vi "CIMAQ_GetPalette.vi"(8 "error in":errorcluster, 11 "Palette Number (gray)":T1(ring)=enum."Full Rainbow") -> (0 "error out":errorcluster, 3 "User Palette":cluster{"Red":u8, "Green":u8, "Blue":u8}[](array[cluster]))   [LabVIEW 2017]
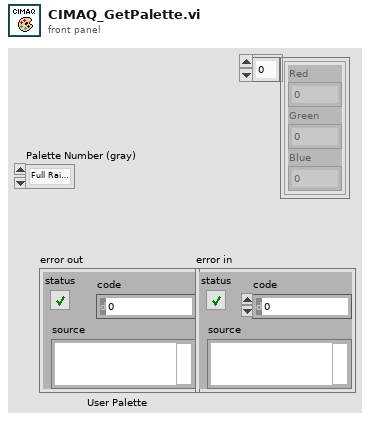
[diagram p1: front panel]
types:
  T1 = enum32{"Gray", "Binary", "Gradient", "Rainbow", "Temperature", "Full Rainbow", "Iron", "Hot Iron", "Hot Metal Blue", "PET"}
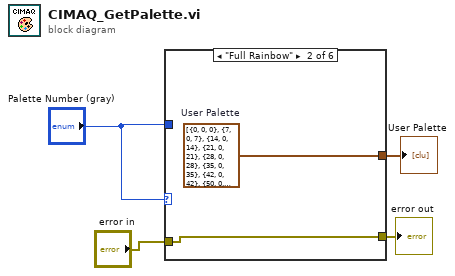
[diagram p0: block diagram]
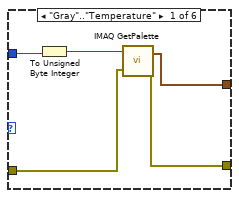
[diagram p2: hidden frame]
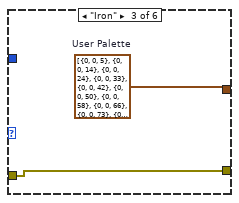
[diagram p3: hidden frame]
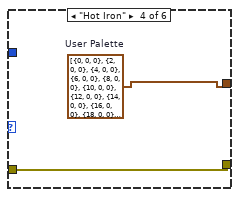
[diagram p4: hidden frame]
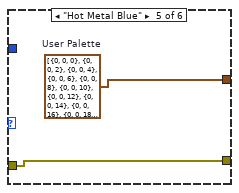
[diagram p5: hidden frame]
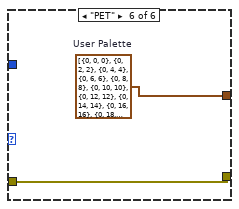
[diagram p6: hidden frame]
diagram:
  n1 = case shown="\"Full Rainbow\"" "Palette Number (gray)" {
    tunnel: "Palette Number (gray)" -> [w9 _ _ _ _ _]
    tunnel: [w7 w11 w13 w14 w17 w18] -> w1
    tunnel: [w6 w10 w12 w15 w16 w19] -> w3
    tunnel: "error in" -> [w5 w10 w12 w15 w16 w19]
    frame "Gray".."Temperature" {
      n2 = To Unsigned Byte Integer(number=w9) -> (unsigned 8bit integer=w8:u8)
      n3 = call "IMAQ GetPalette"("Palette Number (gray)"=w8, "error in (no error)"=w5) -> ("Color Palette"=w7:cluster{"Red":u8, "Green":u8, "Blue":u8}[], "error out"=w6:errorcluster)  [unwired: 3 in]
    }
    frame "Full Rainbow" {
      w11 = cluster{"Red":u8, "Green":u8, "Blue":u8}[] [{"Red"=0, "Green"=0, "Blue"=0}, {"Red"=7, "Green"=0, "Blue"=7}, {"Red"=14, "Green"=0, "Blue"=14}, {"Red"=21, "Green"=0, "Blue"=21}, {"Red"=28, "Green"=0, "Blue"=28}, {"Red"=35, "Green"=0, "Blue"=35}, {"Red"=42, "Green"=0, "Blue"=42}, {"Red"=50, "Green"=0, "Blue"=50}, {"Red"=57, "Green"=0, "Blue"=57}, {"Red"=64, "Green"=0, "Blue"=64}, {"Red"=71, "Green"=0, "Blue"=71}, {"Red"=78, "Green"=0, "Blue"=78}, {"Red"=85, "Green"=0, "Blue"=85}, {"Red"=92, "Green"=0, "Blue"=92}, {"Red"=99, "Green"=0, "Blue"=99}, {"Red"=106, "Green"=0, "Blue"=106}, {"Red"=113, "Green"=0, "Blue"=113}, {"Red"=120, "Green"=0, "Blue"=120}, {"Red"=128, "Green"=0, "Blue"=128}, {"Red"=135, "Green"=0, "Blue"=135}, {"Red"=142, "Green"=0, "Blue"=142}, {"Red"=149, "Green"=0, "Blue"=149}, {"Red"=156, "Green"=0, "Blue"=156}, {"Red"=163, "Green"=0, "Blue"=163}, {"Red"=170, "Green"=0, "Blue"=170}, {"Red"=177, "Green"=0, "Blue"=177}, {"Red"=184, "Green"=0, "Blue"=184}, {"Red"=191, "Green"=0, "Blue"=191}, {"Red"=198, "Green"=0, "Blue"=198}, {"Red"=205, "Green"=0, "Blue"=205}, {"Red"=212, "Green"=0, "Blue"=212}, {"Red"=220, "Green"=0, "Blue"=220}, {"Red"=227, "Green"=0, "Blue"=227}, {"Red"=234, "Green"=0, "Blue"=234}, {"Red"=241, "Green"=0, "Blue"=241}, {"Red"=248, "Green"=0, "Blue"=248}, {"Red"=255, "Green"=0, "Blue"=255}, {"Red"=248, "Green"=0, "Blue"=253}, {"Red"=241, "Green"=0, "Blue"=251}, {"Red"=234, "Green"=0, "Blue"=249}, {"Red"=227, "Green"=0, "Blue"=247}, {"Red"=220, "Green"=0, "Blue"=245}, {"Red"=212, "Green"=0, "Blue"=242}, {"Red"=205, "Green"=0, "Blue"=240}, {"Red"=198, "Green"=0, "Blue"=238}, {"Red"=191, "Green"=0, "Blue"=236}, {"Red"=184, "Green"=0, "Blue"=234}, {"Red"=177, "Green"=0, "Blue"=232}, {"Red"=170, "Green"=0, "Blue"=230}, {"Red"=163, "Green"=0, "Blue"=228}, {"Red"=156, "Green"=0, "Blue"=226}, {"Red"=149, "Green"=0, "Blue"=224}, {"Red"=142, "Green"=0, "Blue"=222}, {"Red"=135, "Green"=0, "Blue"=220}, {"Red"=128, "Green"=0, "Blue"=218}, {"Red"=120, "Green"=0, "Blue"=215}, {"Red"=113, "Green"=0, "Blue"=213}, {"Red"=106, "Green"=0, "Blue"=211}, {"Red"=99, "Green"=0, "Blue"=209}, {"Red"=92, "Green"=0, "Blue"=207}, {"Red"=85, "Green"=0, "Blue"=205}, {"Red"=78, "Green"=0, "Blue"=203}, {"Red"=71, "Green"=0, "Blue"=201}, {"Red"=64, "Green"=0, "Blue"=199}, {"Red"=57, "Green"=0, "Blue"=197}, {"Red"=50, "Green"=0, "Blue"=195}, {"Red"=42, "Green"=0, "Blue"=192}, {"Red"=35, "Green"=0, "Blue"=190}, {"Red"=28, "Green"=0, "Blue"=188}, {"Red"=21, "Green"=0, "Blue"=186}, {"Red"=14, "Green"=0, "Blue"=184}, {"Red"=7, "Green"=0, "Blue"=182}, {"Red"=0, "Green"=0, "Blue"=180}, {"Red"=0, "Green"=7, "Blue"=182}, {"Red"=0, "Green"=14, "Blue"=184}, {"Red"=0, "Green"=21, "Blue"=186}, {"Red"=0, "Green"=28, "Blue"=188}, {"Red"=0, "Green"=35, "Blue"=190}, {"Red"=0, "Green"=42, "Blue"=192}, {"Red"=0, "Green"=50, "Blue"=194}, {"Red"=0, "Green"=57, "Blue"=196}, {"Red"=0, "Green"=64, "Blue"=198}, {"Red"=0, "Green"=71, "Blue"=201}, {"Red"=0, "Green"=78, "Blue"=203}, {"Red"=0, "Green"=85, "Blue"=205}, {"Red"=0, "Green"=92, "Blue"=207}, {"Red"=0, "Green"=99, "Blue"=209}, {"Red"=0, "Green"=106, "Blue"=211}, {"Red"=0, "Green"=113, "Blue"=213}, {"Red"=0, "Green"=120, "Blue"=215}, {"Red"=0, "Green"=128, "Blue"=217}, {"Red"=0, "Green"=135, "Blue"=219}, {"Red"=0, "Green"=142, "Blue"=221}, {"Red"=0, "Green"=149, "Blue"=223}, {"Red"=0, "Green"=156, "Blue"=225}, {"Red"=0, "Green"=163, "Blue"=227}, {"Red"=0, "Green"=170, "Blue"=229}, {"Red"=0, "Green"=177, "Blue"=231}, {"Red"=0, "Green"=184, "Blue"=233}, {"Red"=0, "Green"=191, "Blue"=236}, {"Red"=0, "Green"=198, "Blue"=238}, {"Red"=0, "Green"=205, "Blue"=240}, {"Red"=0, "Green"=213, "Blue"=242}, {"Red"=0, "Green"=220, "Blue"=244}, {"Red"=0, "Green"=227, "Blue"=246}, {"Red"=0, "Green"=234, "Blue"=248}, {"Red"=0, "Green"=241, "Blue"=250}, {"Red"=0, "Green"=248, "Blue"=252}, {"Red"=0, "Green"=255, "Blue"=254}, {"Red"=0, "Green"=253, "Blue"=247}, {"Red"=0, "Green"=251, "Blue"=240}, {"Red"=0, "Green"=250, "Blue"=233}, {"Red"=0, "Green"=248, "Blue"=226}, {"Red"=0, "Green"=246, "Blue"=219}, {"Red"=0, "Green"=244, "Blue"=212}, {"Red"=0, "Green"=242, "Blue"=205}, {"Red"=0, "Green"=241, "Blue"=198}, {"Red"=0, "Green"=239, "Blue"=190}, {"Red"=0, "Green"=237, "Blue"=183}, {"Red"=0, "Green"=235, "Blue"=176}, {"Red"=0, "Green"=233, "Blue"=169}, {"Red"=0, "Green"=232, "Blue"=162}, {"Red"=0, "Green"=230, "Blue"=155}, {"Red"=0, "Green"=228, "Blue"=148}, {"Red"=0, "Green"=226, "Blue"=141}, {"Red"=0, "Green"=224, "Blue"=134}, {"Red"=0, "Green"=222, "Blue"=127}, {"Red"=0, "Green"=221, "Blue"=120}, {"Red"=0, "Green"=219, "Blue"=113}, {"Red"=0, "Green"=217, "Blue"=106}, {"Red"=0, "Green"=215, "Blue"=99}, {"Red"=0, "Green"=213, "Blue"=92}, {"Red"=0, "Green"=212, "Blue"=85}, {"Red"=0, "Green"=210, "Blue"=78}, {"Red"=0, "Green"=208, "Blue"=71}, {"Red"=0, "Green"=206, "Blue"=64}, {"Red"=0, "Green"=204, "Blue"=56}, {"Red"=0, "Green"=203, "Blue"=49}, {"Red"=0, "Green"=201, "Blue"=42}, {"Red"=0, "Green"=199, "Blue"=35}, {"Red"=0, "Green"=197, "Blue"=28}, {"Red"=0, "Green"=195, "Blue"=21}, {"Red"=0, "Green"=194, "Blue"=14}, {"Red"=0, "Green"=192, "Blue"=7}, {"Red"=0, "Green"=190, "Blue"=0}, {"Red"=7, "Green"=192, "Blue"=0}, {"Red"=14, "Green"=194, "Blue"=0}, {"Red"=21, "Green"=195, "Blue"=0}, {"Red"=28, "Green"=197, "Blue"=0}, {"Red"=35, "Green"=199, "Blue"=0}, {"Red"=43, "Green"=201, "Blue"=0}, {"Red"=50, "Green"=202, "Blue"=0}, {"Red"=57, "Green"=204, "Blue"=0}, {"Red"=64, "Green"=206, "Blue"=0}, {"Red"=71, "Green"=208, "Blue"=0}, {"Red"=78, "Green"=210, "Blue"=0}, {"Red"=85, "Green"=211, "Blue"=0}, {"Red"=92, "Green"=213, "Blue"=0}, {"Red"=99, "Green"=215, "Blue"=0}, {"Red"=106, "Green"=217, "Blue"=0}, {"Red"=113, "Green"=218, "Blue"=0}, {"Red"=120, "Green"=220, "Blue"=0}, {"Red"=128, "Green"=222, "Blue"=0}, {"Red"=135, "Green"=224, "Blue"=0}, {"Red"=142, "Green"=226, "Blue"=0}, {"Red"=149, "Green"=227, "Blue"=0}, {"Red"=156, "Green"=229, "Blue"=0}, {"Red"=163, "Green"=231, "Blue"=0}, {"Red"=170, "Green"=233, "Blue"=0}, {"Red"=177, "Green"=234, "Blue"=0}, {"Red"=184, "Green"=236, "Blue"=0}, {"Red"=191, "Green"=238, "Blue"=0}, {"Red"=198, "Green"=240, "Blue"=0}, {"Red"=205, "Green"=242, "Blue"=0}, {"Red"=212, "Green"=243, "Blue"=0}, {"Red"=220, "Green"=245, "Blue"=0}, {"Red"=227, "Green"=247, "Blue"=0}, {"Red"=234, "Green"=249, "Blue"=0}, {"Red"=241, "Green"=250, "Blue"=0}, {"Red"=248, "Green"=252, "Blue"=0}, {"Red"=255, "Green"=254, "Blue"=0}, {"Red"=253, "Green"=247, "Blue"=0}, {"Red"=252, "Green"=240, "Blue"=0}, {"Red"=250, "Green"=233, "Blue"=0}, {"Red"=249, "Green"=226, "Blue"=0}, {"Red"=247, "Green"=219, "Blue"=0}, {"Red"=246, "Green"=212, "Blue"=0}, {"Red"=244, "Green"=205, "Blue"=0}, {"Red"=243, "Green"=198, "Blue"=0}, {"Red"=241, "Green"=190, "Blue"=0}, {"Red"=239, "Green"=183, "Blue"=0}, {"Red"=238, "Green"=176, "Blue"=0}, {"Red"=236, "Green"=169, "Blue"=0}, {"Red"=235, "Green"=162, "Blue"=0}, {"Red"=233, "Green"=155, "Blue"=0}, {"Red"=232, "Green"=148, "Blue"=0}, {"Red"=230, "Green"=141, "Blue"=0}, {"Red"=229, "Green"=134, "Blue"=0}, {"Red"=227, "Green"=127, "Blue"=0}, {"Red"=225, "Green"=120, "Blue"=0}, {"Red"=224, "Green"=113, "Blue"=0}, {"Red"=222, "Green"=106, "Blue"=0}, {"Red"=221, "Green"=99, "Blue"=0}, {"Red"=219, "Green"=92, "Blue"=0}, {"Red"=218, "Green"=85, "Blue"=0}, {"Red"=216, "Green"=78, "Blue"=0}, {"Red"=215, "Green"=71, "Blue"=0}, {"Red"=213, "Green"=64, "Blue"=0}, {"Red"=211, "Green"=56, "Blue"=0}, {"Red"=210, "Green"=49, "Blue"=0}, {"Red"=208, "Green"=42, "Blue"=0}, {"Red"=207, "Green"=35, "Blue"=0}, {"Red"=205, "Green"=28, "Blue"=0}, {"Red"=204, "Green"=21, "Blue"=0}, {"Red"=202, "Green"=14, "Blue"=0}, {"Red"=201, "Green"=7, "Blue"=0}, {"Red"=199, "Green"=0, "Blue"=0}, {"Red"=200, "Green"=7, "Blue"=7}, {"Red"=202, "Green"=13, "Blue"=13}, {"Red"=203, "Green"=20, "Blue"=20}, {"Red"=205, "Green"=26, "Blue"=26}, {"Red"=206, "Green"=33, "Blue"=33}, {"Red"=208, "Green"=39, "Blue"=39}, {"Red"=209, "Green"=46, "Blue"=46}, {"Red"=210, "Green"=52, "Blue"=52}, {"Red"=212, "Green"=59, "Blue"=59}, {"Red"=213, "Green"=65, "Blue"=65}, {"Red"=215, "Green"=72, "Blue"=72}, {"Red"=216, "Green"=78, "Blue"=78}, {"Red"=218, "Green"=85, "Blue"=85}, {"Red"=219, "Green"=92, "Blue"=92}, {"Red"=221, "Green"=98, "Blue"=98}, {"Red"=222, "Green"=105, "Blue"=105}, {"Red"=223, "Green"=111, "Blue"=111}, {"Red"=225, "Green"=118, "Blue"=118}, {"Red"=226, "Green"=124, "Blue"=124}, {"Red"=228, "Green"=131, "Blue"=131}, {"Red"=229, "Green"=137, "Blue"=137}, {"Red"=231, "Green"=144, "Blue"=144}, {"Red"=232, "Green"=150, "Blue"=150}, {"Red"=233, "Green"=157, "Blue"=157}, {"Red"=235, "Green"=163, "Blue"=163}, {"Red"=236, "Green"=170, "Blue"=170}, {"Red"=238, "Green"=177, "Blue"=177}, {"Red"=239, "Green"=183, "Blue"=183}, {"Red"=241, "Green"=190, "Blue"=190}, {"Red"=242, "Green"=196, "Blue"=196}, {"Red"=244, "Green"=203, "Blue"=203}, {"Red"=245, "Green"=209, "Blue"=209}, {"Red"=246, "Green"=216, "Blue"=216}, {"Red"=248, "Green"=222, "Blue"=222}, {"Red"=249, "Green"=229, "Blue"=229}, {"Red"=251, "Green"=235, "Blue"=235}, {"Red"=252, "Green"=242, "Blue"=242}, {"Red"=254, "Green"=248, "Blue"=248}, {"Red"=255, "Green"=255, "Blue"=255}]  # User Palette
    }
    frame "Iron" {
      w13 = cluster{"Red":u8, "Green":u8, "Blue":u8}[] [{"Red"=0, "Green"=0, "Blue"=5}, {"Red"=0, "Green"=0, "Blue"=14}, {"Red"=0, "Green"=0, "Blue"=24}, {"Red"=0, "Green"=0, "Blue"=33}, {"Red"=0, "Green"=0, "Blue"=42}, {"Red"=0, "Green"=0, "Blue"=50}, {"Red"=0, "Green"=0, "Blue"=58}, {"Red"=0, "Green"=0, "Blue"=66}, {"Red"=0, "Green"=0, "Blue"=73}, {"Red"=0, "Green"=0, "Blue"=80}, {"Red"=0, "Green"=0, "Blue"=86}, {"Red"=0, "Green"=0, "Blue"=91}, {"Red"=1, "Green"=0, "Blue"=96}, {"Red"=2, "Green"=0, "Blue"=100}, {"Red"=3, "Green"=0, "Blue"=103}, {"Red"=4, "Green"=0, "Blue"=106}, {"Red"=5, "Green"=0, "Blue"=109}, {"Red"=7, "Green"=0, "Blue"=111}, {"Red"=9, "Green"=0, "Blue"=114}, {"Red"=11, "Green"=0, "Blue"=116}, {"Red"=13, "Green"=0, "Blue"=118}, {"Red"=16, "Green"=0, "Blue"=120}, {"Red"=18, "Green"=0, "Blue"=122}, {"Red"=21, "Green"=0, "Blue"=125}, {"Red"=24, "Green"=0, "Blue"=127}, {"Red"=28, "Green"=0, "Blue"=129}, {"Red"=31, "Green"=0, "Blue"=131}, {"Red"=34, "Green"=0, "Blue"=133}, {"Red"=38, "Green"=0, "Blue"=135}, {"Red"=41, "Green"=0, "Blue"=137}, {"Red"=44, "Green"=0, "Blue"=139}, {"Red"=47, "Green"=0, "Blue"=141}, {"Red"=50, "Green"=0, "Blue"=142}, {"Red"=53, "Green"=0, "Blue"=144}, {"Red"=56, "Green"=0, "Blue"=145}, {"Red"=59, "Green"=0, "Blue"=146}, {"Red"=61, "Green"=0, "Blue"=147}, {"Red"=64, "Green"=0, "Blue"=149}, {"Red"=67, "Green"=0, "Blue"=149}, {"Red"=69, "Green"=0, "Blue"=150}, {"Red"=72, "Green"=0, "Blue"=151}, {"Red"=75, "Green"=0, "Blue"=152}, {"Red"=77, "Green"=0, "Blue"=152}, {"Red"=80, "Green"=0, "Blue"=153}, {"Red"=83, "Green"=0, "Blue"=153}, {"Red"=86, "Green"=0, "Blue"=154}, {"Red"=89, "Green"=0, "Blue"=154}, {"Red"=91, "Green"=0, "Blue"=154}, {"Red"=94, "Green"=0, "Blue"=154}, {"Red"=97, "Green"=0, "Blue"=155}, {"Red"=100, "Green"=0, "Blue"=155}, {"Red"=103, "Green"=0, "Blue"=155}, {"Red"=106, "Green"=0, "Blue"=156}, {"Red"=109, "Green"=0, "Blue"=156}, {"Red"=112, "Green"=0, "Blue"=156}, {"Red"=115, "Green"=0, "Blue"=156}, {"Red"=117, "Green"=0, "Blue"=157}, {"Red"=120, "Green"=0, "Blue"=157}, {"Red"=123, "Green"=0, "Blue"=157}, {"Red"=126, "Green"=0, "Blue"=157}, {"Red"=129, "Green"=0, "Blue"=157}, {"Red"=132, "Green"=0, "Blue"=157}, {"Red"=135, "Green"=0, "Blue"=157}, {"Red"=137, "Green"=0, "Blue"=157}, {"Red"=140, "Green"=0, "Blue"=157}, {"Red"=143, "Green"=0, "Blue"=156}, {"Red"=146, "Green"=0, "Blue"=156}, {"Red"=148, "Green"=0, "Blue"=156}, {"Red"=151, "Green"=0, "Blue"=156}, {"Red"=154, "Green"=0, "Blue"=155}, {"Red"=156, "Green"=0, "Blue"=155}, {"Red"=158, "Green"=0, "Blue"=155}, {"Red"=161, "Green"=0, "Blue"=154}, {"Red"=163, "Green"=0, "Blue"=154}, {"Red"=165, "Green"=0, "Blue"=154}, {"Red"=167, "Green"=0, "Blue"=153}, {"Red"=170, "Green"=0, "Blue"=153}, {"Red"=172, "Green"=0, "Blue"=152}, {"Red"=173, "Green"=0, "Blue"=152}, {"Red"=175, "Green"=0, "Blue"=152}, {"Red"=177, "Green"=0, "Blue"=151}, {"Red"=179, "Green"=0, "Blue"=150}, {"Red"=180, "Green"=1, "Blue"=150}, {"Red"=182, "Green"=1, "Blue"=149}, {"Red"=183, "Green"=2, "Blue"=148}, {"Red"=185, "Green"=2, "Blue"=148}, {"Red"=186, "Green"=3, "Blue"=147}, {"Red"=187, "Green"=4, "Blue"=146}, {"Red"=188, "Green"=4, "Blue"=146}, {"Red"=190, "Green"=5, "Blue"=145}, {"Red"=191, "Green"=6, "Blue"=144}, {"Red"=192, "Green"=7, "Blue"=143}, {"Red"=194, "Green"=8, "Blue"=142}, {"Red"=195, "Green"=9, "Blue"=142}, {"Red"=196, "Green"=10, "Blue"=141}, {"Red"=197, "Green"=11, "Blue"=140}, {"Red"=198, "Green"=13, "Blue"=139}, {"Red"=200, "Green"=14, "Blue"=137}, {"Red"=201, "Green"=15, "Blue"=136}, {"Red"=202, "Green"=17, "Blue"=135}, {"Red"=203, "Green"=18, "Blue"=133}, {"Red"=204, "Green"=20, "Blue"=131}, {"Red"=205, "Green"=21, "Blue"=129}, {"Red"=206, "Green"=23, "Blue"=127}, {"Red"=207, "Green"=24, "Blue"=125}, {"Red"=208, "Green"=26, "Blue"=122}, {"Red"=209, "Green"=28, "Blue"=119}, {"Red"=210, "Green"=30, "Blue"=116}, {"Red"=211, "Green"=31, "Blue"=113}, {"Red"=212, "Green"=33, "Blue"=110}, {"Red"=213, "Green"=35, "Blue"=106}, {"Red"=214, "Green"=37, "Blue"=102}, {"Red"=215, "Green"=39, "Blue"=98}, {"Red"=216, "Green"=40, "Blue"=94}, {"Red"=217, "Green"=42, "Blue"=89}, {"Red"=218, "Green"=44, "Blue"=85}, {"Red"=219, "Green"=46, "Blue"=80}, {"Red"=220, "Green"=48, "Blue"=75}, {"Red"=221, "Green"=49, "Blue"=71}, {"Red"=222, "Green"=51, "Blue"=66}, {"Red"=223, "Green"=53, "Blue"=61}, {"Red"=224, "Green"=55, "Blue"=56}, {"Red"=225, "Green"=57, "Blue"=51}, {"Red"=226, "Green"=58, "Blue"=47}, {"Red"=227, "Green"=60, "Blue"=42}, {"Red"=228, "Green"=62, "Blue"=38}, {"Red"=229, "Green"=64, "Blue"=34}, {"Red"=230, "Green"=66, "Blue"=30}, {"Red"=231, "Green"=67, "Blue"=26}, {"Red"=231, "Green"=69, "Blue"=23}, {"Red"=232, "Green"=71, "Blue"=20}, {"Red"=233, "Green"=73, "Blue"=17}, {"Red"=233, "Green"=75, "Blue"=15}, {"Red"=234, "Green"=77, "Blue"=13}, {"Red"=234, "Green"=78, "Blue"=12}, {"Red"=235, "Green"=80, "Blue"=10}, {"Red"=235, "Green"=82, "Blue"=9}, {"Red"=236, "Green"=84, "Blue"=8}, {"Red"=236, "Green"=86, "Blue"=7}, {"Red"=237, "Green"=87, "Blue"=7}, {"Red"=237, "Green"=89, "Blue"=6}, {"Red"=237, "Green"=91, "Blue"=5}, {"Red"=238, "Green"=92, "Blue"=5}, {"Red"=239, "Green"=94, "Blue"=4}, {"Red"=239, "Green"=95, "Blue"=4}, {"Red"=240, "Green"=97, "Blue"=4}, {"Red"=240, "Green"=98, "Blue"=3}, {"Red"=241, "Green"=100, "Blue"=3}, {"Red"=241, "Green"=101, "Blue"=3}, {"Red"=242, "Green"=102, "Blue"=2}, {"Red"=242, "Green"=104, "Blue"=2}, {"Red"=242, "Green"=106, "Blue"=2}, {"Red"=243, "Green"=107, "Blue"=1}, {"Red"=243, "Green"=109, "Blue"=1}, {"Red"=243, "Green"=111, "Blue"=1}, {"Red"=244, "Green"=112, "Blue"=1}, {"Red"=244, "Green"=114, "Blue"=1}, {"Red"=244, "Green"=116, "Blue"=0}, {"Red"=244, "Green"=117, "Blue"=0}, {"Red"=245, "Green"=119, "Blue"=0}, {"Red"=245, "Green"=121, "Blue"=0}, {"Red"=245, "Green"=123, "Blue"=0}, {"Red"=246, "Green"=125, "Blue"=0}, {"Red"=246, "Green"=126, "Blue"=0}, {"Red"=247, "Green"=128, "Blue"=0}, {"Red"=247, "Green"=130, "Blue"=0}, {"Red"=247, "Green"=132, "Blue"=0}, {"Red"=248, "Green"=134, "Blue"=0}, {"Red"=248, "Green"=135, "Blue"=0}, {"Red"=249, "Green"=137, "Blue"=0}, {"Red"=249, "Green"=139, "Blue"=0}, {"Red"=249, "Green"=141, "Blue"=0}, {"Red"=250, "Green"=143, "Blue"=0}, {"Red"=250, "Green"=145, "Blue"=0}, {"Red"=250, "Green"=147, "Blue"=0}, {"Red"=251, "Green"=148, "Blue"=0}, {"Red"=251, "Green"=150, "Blue"=0}, {"Red"=251, "Green"=152, "Blue"=0}, {"Red"=252, "Green"=154, "Blue"=0}, {"Red"=252, "Green"=156, "Blue"=0}, {"Red"=252, "Green"=158, "Blue"=0}, {"Red"=252, "Green"=160, "Blue"=0}, {"Red"=252, "Green"=162, "Blue"=0}, {"Red"=253, "Green"=164, "Blue"=0}, {"Red"=253, "Green"=166, "Blue"=0}, {"Red"=253, "Green"=167, "Blue"=0}, {"Red"=253, "Green"=169, "Blue"=0}, {"Red"=253, "Green"=171, "Blue"=0}, {"Red"=254, "Green"=173, "Blue"=0}, {"Red"=254, "Green"=175, "Blue"=0}, {"Red"=254, "Green"=177, "Blue"=0}, {"Red"=254, "Green"=179, "Blue"=0}, {"Red"=254, "Green"=181, "Blue"=0}, {"Red"=255, "Green"=183, "Blue"=0}, {"Red"=255, "Green"=185, "Blue"=0}, {"Red"=255, "Green"=187, "Blue"=0}, {"Red"=255, "Green"=189, "Blue"=0}, {"Red"=255, "Green"=191, "Blue"=0}, {"Red"=255, "Green"=192, "Blue"=0}, {"Red"=255, "Green"=194, "Blue"=0}, {"Red"=255, "Green"=196, "Blue"=0}, {"Red"=255, "Green"=198, "Blue"=0}, {"Red"=255, "Green"=199, "Blue"=1}, {"Red"=255, "Green"=201, "Blue"=1}, {"Red"=255, "Green"=203, "Blue"=2}, {"Red"=254, "Green"=204, "Blue"=2}, {"Red"=254, "Green"=206, "Blue"=3}, {"Red"=254, "Green"=208, "Blue"=4}, {"Red"=254, "Green"=209, "Blue"=5}, {"Red"=254, "Green"=211, "Blue"=7}, {"Red"=254, "Green"=212, "Blue"=8}, {"Red"=254, "Green"=213, "Blue"=10}, {"Red"=254, "Green"=215, "Blue"=11}, {"Red"=254, "Green"=216, "Blue"=13}, {"Red"=254, "Green"=218, "Blue"=15}, {"Red"=254, "Green"=219, "Blue"=18}, {"Red"=255, "Green"=221, "Blue"=21}, {"Red"=255, "Green"=222, "Blue"=24}, {"Red"=255, "Green"=223, "Blue"=27}, {"Red"=255, "Green"=225, "Blue"=31}, {"Red"=255, "Green"=226, "Blue"=35}, {"Red"=255, "Green"=227, "Blue"=40}, {"Red"=255, "Green"=229, "Blue"=44}, {"Red"=255, "Green"=230, "Blue"=50}, {"Red"=255, "Green"=231, "Blue"=55}, {"Red"=255, "Green"=233, "Blue"=61}, {"Red"=255, "Green"=234, "Blue"=67}, {"Red"=255, "Green"=235, "Blue"=74}, {"Red"=255, "Green"=236, "Blue"=80}, {"Red"=255, "Green"=237, "Blue"=87}, {"Red"=255, "Green"=238, "Blue"=94}, {"Red"=255, "Green"=239, "Blue"=101}, {"Red"=255, "Green"=240, "Blue"=108}, {"Red"=255, "Green"=240, "Blue"=115}, {"Red"=255, "Green"=241, "Blue"=122}, {"Red"=255, "Green"=242, "Blue"=130}, {"Red"=255, "Green"=243, "Blue"=137}, {"Red"=255, "Green"=243, "Blue"=144}, {"Red"=255, "Green"=244, "Blue"=151}, {"Red"=255, "Green"=244, "Blue"=157}, {"Red"=255, "Green"=245, "Blue"=164}, {"Red"=255, "Green"=246, "Blue"=170}, {"Red"=255, "Green"=246, "Blue"=177}, {"Red"=255, "Green"=247, "Blue"=183}, {"Red"=255, "Green"=248, "Blue"=189}, {"Red"=255, "Green"=248, "Blue"=195}, {"Red"=255, "Green"=249, "Blue"=200}, {"Red"=255, "Green"=250, "Blue"=206}, {"Red"=255, "Green"=251, "Blue"=212}, {"Red"=255, "Green"=251, "Blue"=217}, {"Red"=255, "Green"=252, "Blue"=223}, {"Red"=255, "Green"=253, "Blue"=229}, {"Red"=255, "Green"=253, "Blue"=234}, {"Red"=255, "Green"=254, "Blue"=240}, {"Red"=255, "Green"=255, "Blue"=246}, {"Red"=255, "Green"=255, "Blue"=251}]  # User Palette
    }
    frame "Hot Iron" {
      w14 = cluster{"Red":u8, "Green":u8, "Blue":u8}[] [{"Red"=0, "Green"=0, "Blue"=0}, {"Red"=2, "Green"=0, "Blue"=0}, {"Red"=4, "Green"=0, "Blue"=0}, {"Red"=6, "Green"=0, "Blue"=0}, {"Red"=8, "Green"=0, "Blue"=0}, {"Red"=10, "Green"=0, "Blue"=0}, {"Red"=12, "Green"=0, "Blue"=0}, {"Red"=14, "Green"=0, "Blue"=0}, {"Red"=16, "Green"=0, "Blue"=0}, {"Red"=18, "Green"=0, "Blue"=0}, {"Red"=20, "Green"=0, "Blue"=0}, {"Red"=22, "Green"=0, "Blue"=0}, {"Red"=24, "Green"=0, "Blue"=0}, {"Red"=26, "Green"=0, "Blue"=0}, {"Red"=28, "Green"=0, "Blue"=0}, {"Red"=30, "Green"=0, "Blue"=0}, {"Red"=32, "Green"=0, "Blue"=0}, {"Red"=34, "Green"=0, "Blue"=0}, {"Red"=36, "Green"=0, "Blue"=0}, {"Red"=38, "Green"=0, "Blue"=0}, {"Red"=40, "Green"=0, "Blue"=0}, {"Red"=42, "Green"=0, "Blue"=0}, {"Red"=44, "Green"=0, "Blue"=0}, {"Red"=46, "Green"=0, "Blue"=0}, {"Red"=48, "Green"=0, "Blue"=0}, {"Red"=50, "Green"=0, "Blue"=0}, {"Red"=52, "Green"=0, "Blue"=0}, {"Red"=54, "Green"=0, "Blue"=0}, {"Red"=56, "Green"=0, "Blue"=0}, {"Red"=58, "Green"=0, "Blue"=0}, {"Red"=60, "Green"=0, "Blue"=0}, {"Red"=62, "Green"=0, "Blue"=0}, {"Red"=64, "Green"=0, "Blue"=0}, {"Red"=66, "Green"=0, "Blue"=0}, {"Red"=68, "Green"=0, "Blue"=0}, {"Red"=70, "Green"=0, "Blue"=0}, {"Red"=72, "Green"=0, "Blue"=0}, {"Red"=74, "Green"=0, "Blue"=0}, {"Red"=76, "Green"=0, "Blue"=0}, {"Red"=78, "Green"=0, "Blue"=0}, {"Red"=80, "Green"=0, "Blue"=0}, {"Red"=82, "Green"=0, "Blue"=0}, {"Red"=84, "Green"=0, "Blue"=0}, {"Red"=86, "Green"=0, "Blue"=0}, {"Red"=88, "Green"=0, "Blue"=0}, {"Red"=90, "Green"=0, "Blue"=0}, {"Red"=92, "Green"=0, "Blue"=0}, {"Red"=94, "Green"=0, "Blue"=0}, {"Red"=96, "Green"=0, "Blue"=0}, {"Red"=98, "Green"=0, "Blue"=0}, {"Red"=100, "Green"=0, "Blue"=0}, {"Red"=102, "Green"=0, "Blue"=0}, {"Red"=104, "Green"=0, "Blue"=0}, {"Red"=106, "Green"=0, "Blue"=0}, {"Red"=108, "Green"=0, "Blue"=0}, {"Red"=110, "Green"=0, "Blue"=0}, {"Red"=112, "Green"=0, "Blue"=0}, {"Red"=114, "Green"=0, "Blue"=0}, {"Red"=116, "Green"=0, "Blue"=0}, {"Red"=118, "Green"=0, "Blue"=0}, {"Red"=120, "Green"=0, "Blue"=0}, {"Red"=122, "Green"=0, "Blue"=0}, {"Red"=124, "Green"=0, "Blue"=0}, {"Red"=126, "Green"=0, "Blue"=0}, {"Red"=128, "Green"=0, "Blue"=0}, {"Red"=129, "Green"=0, "Blue"=0}, {"Red"=131, "Green"=0, "Blue"=0}, {"Red"=133, "Green"=0, "Blue"=0}, {"Red"=135, "Green"=0, "Blue"=0}, {"Red"=137, "Green"=0, "Blue"=0}, {"Red"=139, "Green"=0, "Blue"=0}, {"Red"=141, "Green"=0, "Blue"=0}, {"Red"=143, "Green"=0, "Blue"=0}, {"Red"=145, "Green"=0, "Blue"=0}, {"Red"=147, "Green"=0, "Blue"=0}, {"Red"=149, "Green"=0, "Blue"=0}, {"Red"=151, "Green"=0, "Blue"=0}, {"Red"=153, "Green"=0, "Blue"=0}, {"Red"=155, "Green"=0, "Blue"=0}, {"Red"=157, "Green"=0, "Blue"=0}, {"Red"=159, "Green"=0, "Blue"=0}, {"Red"=161, "Green"=0, "Blue"=0}, {"Red"=163, "Green"=0, "Blue"=0}, {"Red"=165, "Green"=0, "Blue"=0}, {"Red"=167, "Green"=0, "Blue"=0}, {"Red"=169, "Green"=0, "Blue"=0}, {"Red"=171, "Green"=0, "Blue"=0}, {"Red"=173, "Green"=0, "Blue"=0}, {"Red"=175, "Green"=0, "Blue"=0}, {"Red"=177, "Green"=0, "Blue"=0}, {"Red"=179, "Green"=0, "Blue"=0}, {"Red"=181, "Green"=0, "Blue"=0}, {"Red"=183, "Green"=0, "Blue"=0}, {"Red"=185, "Green"=0, "Blue"=0}, {"Red"=187, "Green"=0, "Blue"=0}, {"Red"=189, "Green"=0, "Blue"=0}, {"Red"=191, "Green"=0, "Blue"=0}, {"Red"=193, "Green"=0, "Blue"=0}, {"Red"=195, "Green"=0, "Blue"=0}, {"Red"=197, "Green"=0, "Blue"=0}, {"Red"=199, "Green"=0, "Blue"=0}, {"Red"=201, "Green"=0, "Blue"=0}, {"Red"=203, "Green"=0, "Blue"=0}, {"Red"=205, "Green"=0, "Blue"=0}, {"Red"=207, "Green"=0, "Blue"=0}, {"Red"=209, "Green"=0, "Blue"=0}, {"Red"=211, "Green"=0, "Blue"=0}, {"Red"=213, "Green"=0, "Blue"=0}, {"Red"=215, "Green"=0, "Blue"=0}, {"Red"=217, "Green"=0, "Blue"=0}, {"Red"=219, "Green"=0, "Blue"=0}, {"Red"=221, "Green"=0, "Blue"=0}, {"Red"=223, "Green"=0, "Blue"=0}, {"Red"=225, "Green"=0, "Blue"=0}, {"Red"=227, "Green"=0, "Blue"=0}, {"Red"=229, "Green"=0, "Blue"=0}, {"Red"=231, "Green"=0, "Blue"=0}, {"Red"=233, "Green"=0, "Blue"=0}, {"Red"=235, "Green"=0, "Blue"=0}, {"Red"=237, "Green"=0, "Blue"=0}, {"Red"=239, "Green"=0, "Blue"=0}, {"Red"=241, "Green"=0, "Blue"=0}, {"Red"=243, "Green"=0, "Blue"=0}, {"Red"=245, "Green"=0, "Blue"=0}, {"Red"=247, "Green"=0, "Blue"=0}, {"Red"=249, "Green"=0, "Blue"=0}, {"Red"=251, "Green"=0, "Blue"=0}, {"Red"=253, "Green"=0, "Blue"=0}, {"Red"=255, "Green"=0, "Blue"=0}, {"Red"=255, "Green"=2, "Blue"=0}, {"Red"=255, "Green"=4, "Blue"=0}, {"Red"=255, "Green"=6, "Blue"=0}, {"Red"=255, "Green"=8, "Blue"=0}, {"Red"=255, "Green"=10, "Blue"=0}, {"Red"=255, "Green"=12, "Blue"=0}, {"Red"=255, "Green"=14, "Blue"=0}, {"Red"=255, "Green"=16, "Blue"=0}, {"Red"=255, "Green"=18, "Blue"=0}, {"Red"=255, "Green"=20, "Blue"=0}, {"Red"=255, "Green"=22, "Blue"=0}, {"Red"=255, "Green"=24, "Blue"=0}, {"Red"=255, "Green"=26, "Blue"=0}, {"Red"=255, "Green"=28, "Blue"=0}, {"Red"=255, "Green"=30, "Blue"=0}, {"Red"=255, "Green"=32, "Blue"=0}, {"Red"=255, "Green"=34, "Blue"=0}, {"Red"=255, "Green"=36, "Blue"=0}, {"Red"=255, "Green"=38, "Blue"=0}, {"Red"=255, "Green"=40, "Blue"=0}, {"Red"=255, "Green"=42, "Blue"=0}, {"Red"=255, "Green"=44, "Blue"=0}, {"Red"=255, "Green"=46, "Blue"=0}, {"Red"=255, "Green"=48, "Blue"=0}, {"Red"=255, "Green"=50, "Blue"=0}, {"Red"=255, "Green"=52, "Blue"=0}, {"Red"=255, "Green"=54, "Blue"=0}, {"Red"=255, "Green"=56, "Blue"=0}, {"Red"=255, "Green"=58, "Blue"=0}, {"Red"=255, "Green"=60, "Blue"=0}, {"Red"=255, "Green"=62, "Blue"=0}, {"Red"=255, "Green"=64, "Blue"=0}, {"Red"=255, "Green"=66, "Blue"=0}, {"Red"=255, "Green"=68, "Blue"=0}, {"Red"=255, "Green"=70, "Blue"=0}, {"Red"=255, "Green"=72, "Blue"=0}, {"Red"=255, "Green"=74, "Blue"=0}, {"Red"=255, "Green"=76, "Blue"=0}, {"Red"=255, "Green"=78, "Blue"=0}, {"Red"=255, "Green"=80, "Blue"=0}, {"Red"=255, "Green"=82, "Blue"=0}, {"Red"=255, "Green"=84, "Blue"=0}, {"Red"=255, "Green"=86, "Blue"=0}, {"Red"=255, "Green"=88, "Blue"=0}, {"Red"=255, "Green"=90, "Blue"=0}, {"Red"=255, "Green"=92, "Blue"=0}, {"Red"=255, "Green"=94, "Blue"=0}, {"Red"=255, "Green"=96, "Blue"=0}, {"Red"=255, "Green"=98, "Blue"=0}, {"Red"=255, "Green"=100, "Blue"=0}, {"Red"=255, "Green"=102, "Blue"=0}, {"Red"=255, "Green"=104, "Blue"=0}, {"Red"=255, "Green"=106, "Blue"=0}, {"Red"=255, "Green"=108, "Blue"=0}, {"Red"=255, "Green"=110, "Blue"=0}, {"Red"=255, "Green"=112, "Blue"=0}, {"Red"=255, "Green"=114, "Blue"=0}, {"Red"=255, "Green"=116, "Blue"=0}, {"Red"=255, "Green"=118, "Blue"=0}, {"Red"=255, "Green"=120, "Blue"=0}, {"Red"=255, "Green"=122, "Blue"=0}, {"Red"=255, "Green"=124, "Blue"=0}, {"Red"=255, "Green"=126, "Blue"=0}, {"Red"=255, "Green"=128, "Blue"=4}, {"Red"=255, "Green"=130, "Blue"=8}, {"Red"=255, "Green"=132, "Blue"=12}, {"Red"=255, "Green"=134, "Blue"=16}, {"Red"=255, "Green"=136, "Blue"=20}, {"Red"=255, "Green"=138, "Blue"=24}, {"Red"=255, "Green"=140, "Blue"=28}, {"Red"=255, "Green"=142, "Blue"=32}, {"Red"=255, "Green"=144, "Blue"=36}, {"Red"=255, "Green"=146, "Blue"=40}, {"Red"=255, "Green"=148, "Blue"=44}, {"Red"=255, "Green"=150, "Blue"=48}, {"Red"=255, "Green"=152, "Blue"=52}, {"Red"=255, "Green"=154, "Blue"=56}, {"Red"=255, "Green"=156, "Blue"=60}, {"Red"=255, "Green"=158, "Blue"=64}, {"Red"=255, "Green"=160, "Blue"=68}, {"Red"=255, "Green"=162, "Blue"=72}, {"Red"=255, "Green"=164, "Blue"=76}, {"Red"=255, "Green"=166, "Blue"=80}, {"Red"=255, "Green"=168, "Blue"=84}, {"Red"=255, "Green"=170, "Blue"=88}, {"Red"=255, "Green"=172, "Blue"=92}, {"Red"=255, "Green"=174, "Blue"=96}, {"Red"=255, "Green"=176, "Blue"=100}, {"Red"=255, "Green"=178, "Blue"=104}, {"Red"=255, "Green"=180, "Blue"=108}, {"Red"=255, "Green"=182, "Blue"=112}, {"Red"=255, "Green"=184, "Blue"=116}, {"Red"=255, "Green"=186, "Blue"=120}, {"Red"=255, "Green"=188, "Blue"=124}, {"Red"=255, "Green"=190, "Blue"=128}, {"Red"=255, "Green"=193, "Blue"=131}, {"Red"=255, "Green"=195, "Blue"=135}, {"Red"=255, "Green"=197, "Blue"=139}, {"Red"=255, "Green"=199, "Blue"=143}, {"Red"=255, "Green"=201, "Blue"=147}, {"Red"=255, "Green"=203, "Blue"=151}, {"Red"=255, "Green"=205, "Blue"=155}, {"Red"=255, "Green"=207, "Blue"=159}, {"Red"=255, "Green"=209, "Blue"=163}, {"Red"=255, "Green"=211, "Blue"=167}, {"Red"=255, "Green"=213, "Blue"=171}, {"Red"=255, "Green"=215, "Blue"=175}, {"Red"=255, "Green"=217, "Blue"=179}, {"Red"=255, "Green"=219, "Blue"=183}, {"Red"=255, "Green"=221, "Blue"=187}, {"Red"=255, "Green"=223, "Blue"=191}, {"Red"=255, "Green"=225, "Blue"=195}, {"Red"=255, "Green"=227, "Blue"=199}, {"Red"=255, "Green"=229, "Blue"=203}, {"Red"=255, "Green"=231, "Blue"=207}, {"Red"=255, "Green"=233, "Blue"=211}, {"Red"=255, "Green"=235, "Blue"=215}, {"Red"=255, "Green"=237, "Blue"=219}, {"Red"=255, "Green"=239, "Blue"=223}, {"Red"=255, "Green"=241, "Blue"=227}, {"Red"=255, "Green"=243, "Blue"=231}, {"Red"=255, "Green"=245, "Blue"=235}, {"Red"=255, "Green"=247, "Blue"=239}, {"Red"=255, "Green"=249, "Blue"=243}, {"Red"=255, "Green"=251, "Blue"=247}, {"Red"=255, "Green"=253, "Blue"=251}, {"Red"=255, "Green"=255, "Blue"=255}]  # User Palette
    }
    frame "Hot Metal Blue" {
      w17 = cluster{"Red":u8, "Green":u8, "Blue":u8}[] [{"Red"=0, "Green"=0, "Blue"=0}, {"Red"=0, "Green"=0, "Blue"=2}, {"Red"=0, "Green"=0, "Blue"=4}, {"Red"=0, "Green"=0, "Blue"=6}, {"Red"=0, "Green"=0, "Blue"=8}, {"Red"=0, "Green"=0, "Blue"=10}, {"Red"=0, "Green"=0, "Blue"=12}, {"Red"=0, "Green"=0, "Blue"=14}, {"Red"=0, "Green"=0, "Blue"=16}, {"Red"=0, "Green"=0, "Blue"=18}, {"Red"=0, "Green"=0, "Blue"=20}, {"Red"=0, "Green"=0, "Blue"=22}, {"Red"=0, "Green"=0, "Blue"=24}, {"Red"=0, "Green"=0, "Blue"=26}, {"Red"=0, "Green"=0, "Blue"=28}, {"Red"=0, "Green"=0, "Blue"=29}, {"Red"=0, "Green"=0, "Blue"=31}, {"Red"=0, "Green"=0, "Blue"=33}, {"Red"=0, "Green"=0, "Blue"=35}, {"Red"=0, "Green"=0, "Blue"=37}, {"Red"=0, "Green"=0, "Blue"=39}, {"Red"=0, "Green"=0, "Blue"=41}, {"Red"=0, "Green"=0, "Blue"=43}, {"Red"=0, "Green"=0, "Blue"=45}, {"Red"=0, "Green"=0, "Blue"=47}, {"Red"=0, "Green"=0, "Blue"=49}, {"Red"=0, "Green"=0, "Blue"=51}, {"Red"=0, "Green"=0, "Blue"=53}, {"Red"=0, "Green"=0, "Blue"=55}, {"Red"=0, "Green"=0, "Blue"=57}, {"Red"=0, "Green"=0, "Blue"=59}, {"Red"=0, "Green"=0, "Blue"=61}, {"Red"=0, "Green"=0, "Blue"=63}, {"Red"=0, "Green"=0, "Blue"=65}, {"Red"=0, "Green"=0, "Blue"=67}, {"Red"=0, "Green"=0, "Blue"=69}, {"Red"=0, "Green"=0, "Blue"=71}, {"Red"=0, "Green"=0, "Blue"=73}, {"Red"=0, "Green"=0, "Blue"=75}, {"Red"=0, "Green"=0, "Blue"=77}, {"Red"=0, "Green"=0, "Blue"=79}, {"Red"=0, "Green"=0, "Blue"=81}, {"Red"=0, "Green"=0, "Blue"=83}, {"Red"=0, "Green"=0, "Blue"=84}, {"Red"=0, "Green"=0, "Blue"=86}, {"Red"=0, "Green"=0, "Blue"=88}, {"Red"=0, "Green"=0, "Blue"=90}, {"Red"=0, "Green"=0, "Blue"=92}, {"Red"=0, "Green"=0, "Blue"=94}, {"Red"=0, "Green"=0, "Blue"=96}, {"Red"=0, "Green"=0, "Blue"=98}, {"Red"=0, "Green"=0, "Blue"=100}, {"Red"=0, "Green"=0, "Blue"=102}, {"Red"=0, "Green"=0, "Blue"=104}, {"Red"=0, "Green"=0, "Blue"=106}, {"Red"=0, "Green"=0, "Blue"=108}, {"Red"=0, "Green"=0, "Blue"=110}, {"Red"=0, "Green"=0, "Blue"=112}, {"Red"=0, "Green"=0, "Blue"=114}, {"Red"=0, "Green"=0, "Blue"=116}, {"Red"=0, "Green"=0, "Blue"=118}, {"Red"=0, "Green"=0, "Blue"=120}, {"Red"=0, "Green"=0, "Blue"=122}, {"Red"=0, "Green"=0, "Blue"=124}, {"Red"=0, "Green"=0, "Blue"=126}, {"Red"=0, "Green"=0, "Blue"=128}, {"Red"=0, "Green"=0, "Blue"=130}, {"Red"=0, "Green"=0, "Blue"=132}, {"Red"=0, "Green"=0, "Blue"=134}, {"Red"=0, "Green"=0, "Blue"=136}, {"Red"=0, "Green"=0, "Blue"=138}, {"Red"=0, "Green"=0, "Blue"=139}, {"Red"=0, "Green"=0, "Blue"=141}, {"Red"=0, "Green"=0, "Blue"=143}, {"Red"=0, "Green"=0, "Blue"=145}, {"Red"=0, "Green"=0, "Blue"=147}, {"Red"=0, "Green"=0, "Blue"=149}, {"Red"=0, "Green"=0, "Blue"=151}, {"Red"=0, "Green"=0, "Blue"=153}, {"Red"=0, "Green"=0, "Blue"=155}, {"Red"=0, "Green"=0, "Blue"=157}, {"Red"=0, "Green"=0, "Blue"=159}, {"Red"=0, "Green"=0, "Blue"=161}, {"Red"=0, "Green"=0, "Blue"=163}, {"Red"=0, "Green"=0, "Blue"=165}, {"Red"=0, "Green"=0, "Blue"=167}, {"Red"=3, "Green"=0, "Blue"=169}, {"Red"=6, "Green"=0, "Blue"=171}, {"Red"=9, "Green"=0, "Blue"=173}, {"Red"=12, "Green"=0, "Blue"=175}, {"Red"=15, "Green"=0, "Blue"=177}, {"Red"=18, "Green"=0, "Blue"=179}, {"Red"=21, "Green"=0, "Blue"=181}, {"Red"=24, "Green"=0, "Blue"=183}, {"Red"=26, "Green"=0, "Blue"=184}, {"Red"=29, "Green"=0, "Blue"=186}, {"Red"=32, "Green"=0, "Blue"=188}, {"Red"=35, "Green"=0, "Blue"=190}, {"Red"=38, "Green"=0, "Blue"=192}, {"Red"=41, "Green"=0, "Blue"=194}, {"Red"=44, "Green"=0, "Blue"=196}, {"Red"=47, "Green"=0, "Blue"=198}, {"Red"=50, "Green"=0, "Blue"=200}, {"Red"=52, "Green"=0, "Blue"=197}, {"Red"=55, "Green"=0, "Blue"=194}, {"Red"=57, "Green"=0, "Blue"=191}, {"Red"=59, "Green"=0, "Blue"=188}, {"Red"=62, "Green"=0, "Blue"=185}, {"Red"=64, "Green"=0, "Blue"=182}, {"Red"=66, "Green"=0, "Blue"=179}, {"Red"=69, "Green"=0, "Blue"=176}, {"Red"=71, "Green"=0, "Blue"=174}, {"Red"=74, "Green"=0, "Blue"=171}, {"Red"=76, "Green"=0, "Blue"=168}, {"Red"=78, "Green"=0, "Blue"=165}, {"Red"=81, "Green"=0, "Blue"=162}, {"Red"=83, "Green"=0, "Blue"=159}, {"Red"=85, "Green"=0, "Blue"=156}, {"Red"=88, "Green"=0, "Blue"=153}, {"Red"=90, "Green"=0, "Blue"=150}, {"Red"=93, "Green"=2, "Blue"=144}, {"Red"=96, "Green"=4, "Blue"=138}, {"Red"=99, "Green"=6, "Blue"=132}, {"Red"=102, "Green"=8, "Blue"=126}, {"Red"=105, "Green"=9, "Blue"=121}, {"Red"=108, "Green"=11, "Blue"=115}, {"Red"=111, "Green"=13, "Blue"=109}, {"Red"=114, "Green"=15, "Blue"=103}, {"Red"=116, "Green"=17, "Blue"=97}, {"Red"=119, "Green"=19, "Blue"=91}, {"Red"=122, "Green"=21, "Blue"=85}, {"Red"=125, "Green"=23, "Blue"=79}, {"Red"=128, "Green"=24, "Blue"=74}, {"Red"=131, "Green"=26, "Blue"=68}, {"Red"=134, "Green"=28, "Blue"=62}, {"Red"=137, "Green"=30, "Blue"=56}, {"Red"=140, "Green"=32, "Blue"=50}, {"Red"=143, "Green"=34, "Blue"=47}, {"Red"=146, "Green"=36, "Blue"=44}, {"Red"=149, "Green"=38, "Blue"=41}, {"Red"=152, "Green"=40, "Blue"=38}, {"Red"=155, "Green"=41, "Blue"=35}, {"Red"=158, "Green"=43, "Blue"=32}, {"Red"=161, "Green"=45, "Blue"=29}, {"Red"=164, "Green"=47, "Blue"=26}, {"Red"=166, "Green"=49, "Blue"=24}, {"Red"=169, "Green"=51, "Blue"=21}, {"Red"=172, "Green"=53, "Blue"=18}, {"Red"=175, "Green"=55, "Blue"=15}, {"Red"=178, "Green"=56, "Blue"=12}, {"Red"=181, "Green"=58, "Blue"=9}, {"Red"=184, "Green"=60, "Blue"=6}, {"Red"=187, "Green"=62, "Blue"=3}, {"Red"=190, "Green"=64, "Blue"=0}, {"Red"=194, "Green"=66, "Blue"=0}, {"Red"=198, "Green"=68, "Blue"=0}, {"Red"=201, "Green"=70, "Blue"=0}, {"Red"=205, "Green"=72, "Blue"=0}, {"Red"=209, "Green"=73, "Blue"=0}, {"Red"=213, "Green"=75, "Blue"=0}, {"Red"=217, "Green"=77, "Blue"=0}, {"Red"=221, "Green"=79, "Blue"=0}, {"Red"=224, "Green"=81, "Blue"=0}, {"Red"=228, "Green"=83, "Blue"=0}, {"Red"=232, "Green"=85, "Blue"=0}, {"Red"=236, "Green"=87, "Blue"=0}, {"Red"=240, "Green"=88, "Blue"=0}, {"Red"=244, "Green"=90, "Blue"=0}, {"Red"=247, "Green"=92, "Blue"=0}, {"Red"=251, "Green"=94, "Blue"=0}, {"Red"=255, "Green"=96, "Blue"=0}, {"Red"=255, "Green"=98, "Blue"=3}, {"Red"=255, "Green"=100, "Blue"=6}, {"Red"=255, "Green"=102, "Blue"=9}, {"Red"=255, "Green"=103, "Blue"=12}, {"Red"=255, "Green"=105, "Blue"=15}, {"Red"=255, "Green"=107, "Blue"=18}, {"Red"=255, "Green"=109, "Blue"=21}, {"Red"=255, "Green"=111, "Blue"=24}, {"Red"=255, "Green"=113, "Blue"=27}, {"Red"=255, "Green"=115, "Blue"=30}, {"Red"=255, "Green"=117, "Blue"=33}, {"Red"=255, "Green"=118, "Blue"=36}, {"Red"=255, "Green"=120, "Blue"=39}, {"Red"=255, "Green"=122, "Blue"=42}, {"Red"=255, "Green"=124, "Blue"=45}, {"Red"=255, "Green"=126, "Blue"=48}, {"Red"=255, "Green"=128, "Blue"=51}, {"Red"=255, "Green"=130, "Blue"=54}, {"Red"=255, "Green"=132, "Blue"=57}, {"Red"=255, "Green"=133, "Blue"=60}, {"Red"=255, "Green"=135, "Blue"=63}, {"Red"=255, "Green"=137, "Blue"=66}, {"Red"=255, "Green"=139, "Blue"=69}, {"Red"=255, "Green"=141, "Blue"=72}, {"Red"=255, "Green"=143, "Blue"=75}, {"Red"=255, "Green"=145, "Blue"=78}, {"Red"=255, "Green"=147, "Blue"=81}, {"Red"=255, "Green"=148, "Blue"=84}, {"Red"=255, "Green"=150, "Blue"=87}, {"Red"=255, "Green"=152, "Blue"=90}, {"Red"=255, "Green"=154, "Blue"=93}, {"Red"=255, "Green"=156, "Blue"=96}, {"Red"=255, "Green"=158, "Blue"=99}, {"Red"=255, "Green"=160, "Blue"=102}, {"Red"=255, "Green"=161, "Blue"=105}, {"Red"=255, "Green"=163, "Blue"=108}, {"Red"=255, "Green"=165, "Blue"=111}, {"Red"=255, "Green"=167, "Blue"=114}, {"Red"=255, "Green"=169, "Blue"=117}, {"Red"=255, "Green"=171, "Blue"=120}, {"Red"=255, "Green"=173, "Blue"=123}, {"Red"=255, "Green"=175, "Blue"=126}, {"Red"=255, "Green"=176, "Blue"=129}, {"Red"=255, "Green"=178, "Blue"=132}, {"Red"=255, "Green"=180, "Blue"=135}, {"Red"=255, "Green"=182, "Blue"=138}, {"Red"=255, "Green"=184, "Blue"=141}, {"Red"=255, "Green"=186, "Blue"=144}, {"Red"=255, "Green"=188, "Blue"=147}, {"Red"=255, "Green"=190, "Blue"=150}, {"Red"=255, "Green"=191, "Blue"=153}, {"Red"=255, "Green"=193, "Blue"=156}, {"Red"=255, "Green"=195, "Blue"=159}, {"Red"=255, "Green"=197, "Blue"=162}, {"Red"=255, "Green"=199, "Blue"=165}, {"Red"=255, "Green"=201, "Blue"=168}, {"Red"=255, "Green"=203, "Blue"=171}, {"Red"=255, "Green"=204, "Blue"=174}, {"Red"=255, "Green"=206, "Blue"=177}, {"Red"=255, "Green"=208, "Blue"=180}, {"Red"=255, "Green"=210, "Blue"=183}, {"Red"=255, "Green"=212, "Blue"=186}, {"Red"=255, "Green"=214, "Blue"=189}, {"Red"=255, "Green"=216, "Blue"=192}, {"Red"=255, "Green"=218, "Blue"=195}, {"Red"=255, "Green"=219, "Blue"=198}, {"Red"=255, "Green"=221, "Blue"=201}, {"Red"=255, "Green"=223, "Blue"=204}, {"Red"=255, "Green"=225, "Blue"=207}, {"Red"=255, "Green"=227, "Blue"=210}, {"Red"=255, "Green"=229, "Blue"=213}, {"Red"=255, "Green"=231, "Blue"=216}, {"Red"=255, "Green"=233, "Blue"=219}, {"Red"=255, "Green"=234, "Blue"=222}, {"Red"=255, "Green"=236, "Blue"=225}, {"Red"=255, "Green"=238, "Blue"=228}, {"Red"=255, "Green"=240, "Blue"=231}, {"Red"=255, "Green"=242, "Blue"=234}, {"Red"=255, "Green"=244, "Blue"=237}, {"Red"=255, "Green"=246, "Blue"=240}, {"Red"=255, "Green"=248, "Blue"=243}, {"Red"=255, "Green"=249, "Blue"=246}, {"Red"=255, "Green"=251, "Blue"=249}, {"Red"=255, "Green"=253, "Blue"=252}, {"Red"=255, "Green"=255, "Blue"=255}]  # User Palette
    }
    frame "PET" {
      w18 = cluster{"Red":u8, "Green":u8, "Blue":u8}[] [{"Red"=0, "Green"=0, "Blue"=0}, {"Red"=0, "Green"=2, "Blue"=2}, {"Red"=0, "Green"=4, "Blue"=4}, {"Red"=0, "Green"=6, "Blue"=6}, {"Red"=0, "Green"=8, "Blue"=8}, {"Red"=0, "Green"=10, "Blue"=10}, {"Red"=0, "Green"=12, "Blue"=12}, {"Red"=0, "Green"=14, "Blue"=14}, {"Red"=0, "Green"=16, "Blue"=16}, {"Red"=0, "Green"=18, "Blue"=18}, {"Red"=0, "Green"=20, "Blue"=20}, {"Red"=0, "Green"=22, "Blue"=22}, {"Red"=0, "Green"=24, "Blue"=24}, {"Red"=0, "Green"=26, "Blue"=26}, {"Red"=0, "Green"=28, "Blue"=28}, {"Red"=0, "Green"=30, "Blue"=30}, {"Red"=0, "Green"=33, "Blue"=32}, {"Red"=0, "Green"=35, "Blue"=34}, {"Red"=0, "Green"=37, "Blue"=36}, {"Red"=0, "Green"=39, "Blue"=38}, {"Red"=0, "Green"=41, "Blue"=40}, {"Red"=0, "Green"=43, "Blue"=42}, {"Red"=0, "Green"=45, "Blue"=44}, {"Red"=0, "Green"=47, "Blue"=46}, {"Red"=0, "Green"=49, "Blue"=48}, {"Red"=0, "Green"=51, "Blue"=50}, {"Red"=0, "Green"=53, "Blue"=52}, {"Red"=0, "Green"=55, "Blue"=54}, {"Red"=0, "Green"=57, "Blue"=56}, {"Red"=0, "Green"=59, "Blue"=58}, {"Red"=0, "Green"=61, "Blue"=60}, {"Red"=0, "Green"=63, "Blue"=62}, {"Red"=0, "Green"=65, "Blue"=63}, {"Red"=0, "Green"=67, "Blue"=65}, {"Red"=0, "Green"=69, "Blue"=67}, {"Red"=0, "Green"=71, "Blue"=69}, {"Red"=0, "Green"=73, "Blue"=71}, {"Red"=0, "Green"=75, "Blue"=73}, {"Red"=0, "Green"=77, "Blue"=75}, {"Red"=0, "Green"=79, "Blue"=77}, {"Red"=0, "Green"=81, "Blue"=79}, {"Red"=0, "Green"=83, "Blue"=81}, {"Red"=0, "Green"=85, "Blue"=83}, {"Red"=0, "Green"=87, "Blue"=85}, {"Red"=0, "Green"=89, "Blue"=87}, {"Red"=0, "Green"=91, "Blue"=89}, {"Red"=0, "Green"=93, "Blue"=91}, {"Red"=0, "Green"=95, "Blue"=93}, {"Red"=0, "Green"=98, "Blue"=95}, {"Red"=0, "Green"=100, "Blue"=97}, {"Red"=0, "Green"=102, "Blue"=99}, {"Red"=0, "Green"=104, "Blue"=101}, {"Red"=0, "Green"=106, "Blue"=103}, {"Red"=0, "Green"=108, "Blue"=105}, {"Red"=0, "Green"=110, "Blue"=107}, {"Red"=0, "Green"=112, "Blue"=109}, {"Red"=0, "Green"=114, "Blue"=111}, {"Red"=0, "Green"=116, "Blue"=113}, {"Red"=0, "Green"=118, "Blue"=115}, {"Red"=0, "Green"=120, "Blue"=117}, {"Red"=0, "Green"=122, "Blue"=119}, {"Red"=0, "Green"=124, "Blue"=121}, {"Red"=0, "Green"=126, "Blue"=123}, {"Red"=0, "Green"=128, "Blue"=125}, {"Red"=2, "Green"=126, "Blue"=127}, {"Red"=4, "Green"=124, "Blue"=129}, {"Red"=6, "Green"=122, "Blue"=131}, {"Red"=8, "Green"=120, "Blue"=133}, {"Red"=10, "Green"=118, "Blue"=135}, {"Red"=12, "Green"=116, "Blue"=137}, {"Red"=14, "Green"=114, "Blue"=139}, {"Red"=16, "Green"=112, "Blue"=141}, {"Red"=18, "Green"=110, "Blue"=143}, {"Red"=20, "Green"=108, "Blue"=145}, {"Red"=22, "Green"=106, "Blue"=147}, {"Red"=24, "Green"=104, "Blue"=149}, {"Red"=26, "Green"=102, "Blue"=151}, {"Red"=28, "Green"=100, "Blue"=153}, {"Red"=30, "Green"=98, "Blue"=155}, {"Red"=32, "Green"=96, "Blue"=157}, {"Red"=33, "Green"=95, "Blue"=159}, {"Red"=35, "Green"=93, "Blue"=161}, {"Red"=37, "Green"=91, "Blue"=163}, {"Red"=39, "Green"=89, "Blue"=165}, {"Red"=41, "Green"=87, "Blue"=167}, {"Red"=43, "Green"=85, "Blue"=169}, {"Red"=45, "Green"=83, "Blue"=171}, {"Red"=47, "Green"=81, "Blue"=173}, {"Red"=49, "Green"=79, "Blue"=175}, {"Red"=51, "Green"=77, "Blue"=177}, {"Red"=53, "Green"=75, "Blue"=179}, {"Red"=55, "Green"=73, "Blue"=181}, {"Red"=57, "Green"=71, "Blue"=183}, {"Red"=59, "Green"=69, "Blue"=185}, {"Red"=61, "Green"=67, "Blue"=187}, {"Red"=63, "Green"=65, "Blue"=189}, {"Red"=65, "Green"=63, "Blue"=191}, {"Red"=67, "Green"=61, "Blue"=193}, {"Red"=69, "Green"=59, "Blue"=195}, {"Red"=71, "Green"=57, "Blue"=197}, {"Red"=73, "Green"=55, "Blue"=199}, {"Red"=75, "Green"=53, "Blue"=201}, {"Red"=77, "Green"=51, "Blue"=203}, {"Red"=79, "Green"=49, "Blue"=205}, {"Red"=81, "Green"=47, "Blue"=207}, {"Red"=83, "Green"=45, "Blue"=209}, {"Red"=85, "Green"=43, "Blue"=211}, {"Red"=87, "Green"=41, "Blue"=213}, {"Red"=89, "Green"=39, "Blue"=215}, {"Red"=91, "Green"=37, "Blue"=217}, {"Red"=93, "Green"=35, "Blue"=219}, {"Red"=95, "Green"=33, "Blue"=221}, {"Red"=96, "Green"=32, "Blue"=223}, {"Red"=98, "Green"=30, "Blue"=225}, {"Red"=100, "Green"=28, "Blue"=227}, {"Red"=102, "Green"=26, "Blue"=229}, {"Red"=104, "Green"=24, "Blue"=231}, {"Red"=106, "Green"=22, "Blue"=233}, {"Red"=108, "Green"=20, "Blue"=235}, {"Red"=110, "Green"=18, "Blue"=237}, {"Red"=112, "Green"=16, "Blue"=239}, {"Red"=114, "Green"=14, "Blue"=241}, {"Red"=116, "Green"=12, "Blue"=243}, {"Red"=118, "Green"=10, "Blue"=245}, {"Red"=120, "Green"=8, "Blue"=247}, {"Red"=122, "Green"=6, "Blue"=249}, {"Red"=124, "Green"=4, "Blue"=251}, {"Red"=126, "Green"=2, "Blue"=253}, {"Red"=128, "Green"=0, "Blue"=255}, {"Red"=130, "Green"=2, "Blue"=251}, {"Red"=132, "Green"=4, "Blue"=247}, {"Red"=134, "Green"=6, "Blue"=243}, {"Red"=136, "Green"=8, "Blue"=239}, {"Red"=138, "Green"=10, "Blue"=235}, {"Red"=140, "Green"=12, "Blue"=231}, {"Red"=142, "Green"=14, "Blue"=227}, {"Red"=144, "Green"=16, "Blue"=223}, {"Red"=146, "Green"=18, "Blue"=219}, {"Red"=148, "Green"=20, "Blue"=215}, {"Red"=150, "Green"=22, "Blue"=211}, {"Red"=152, "Green"=24, "Blue"=207}, {"Red"=154, "Green"=26, "Blue"=203}, {"Red"=156, "Green"=28, "Blue"=199}, {"Red"=158, "Green"=30, "Blue"=195}, {"Red"=160, "Green"=32, "Blue"=191}, {"Red"=162, "Green"=34, "Blue"=187}, {"Red"=164, "Green"=36, "Blue"=183}, {"Red"=166, "Green"=38, "Blue"=179}, {"Red"=168, "Green"=40, "Blue"=175}, {"Red"=170, "Green"=42, "Blue"=171}, {"Red"=172, "Green"=44, "Blue"=167}, {"Red"=174, "Green"=46, "Blue"=163}, {"Red"=176, "Green"=48, "Blue"=159}, {"Red"=178, "Green"=50, "Blue"=155}, {"Red"=180, "Green"=52, "Blue"=151}, {"Red"=182, "Green"=54, "Blue"=147}, {"Red"=184, "Green"=56, "Blue"=143}, {"Red"=186, "Green"=58, "Blue"=139}, {"Red"=188, "Green"=60, "Blue"=135}, {"Red"=190, "Green"=62, "Blue"=131}, {"Red"=192, "Green"=64, "Blue"=128}, {"Red"=193, "Green"=66, "Blue"=124}, {"Red"=195, "Green"=68, "Blue"=120}, {"Red"=197, "Green"=70, "Blue"=116}, {"Red"=199, "Green"=72, "Blue"=112}, {"Red"=201, "Green"=74, "Blue"=108}, {"Red"=203, "Green"=76, "Blue"=104}, {"Red"=205, "Green"=78, "Blue"=100}, {"Red"=207, "Green"=80, "Blue"=96}, {"Red"=209, "Green"=82, "Blue"=92}, {"Red"=211, "Green"=84, "Blue"=88}, {"Red"=213, "Green"=86, "Blue"=84}, {"Red"=215, "Green"=88, "Blue"=80}, {"Red"=217, "Green"=90, "Blue"=76}, {"Red"=219, "Green"=92, "Blue"=72}, {"Red"=221, "Green"=94, "Blue"=68}, {"Red"=223, "Green"=96, "Blue"=64}, {"Red"=225, "Green"=98, "Blue"=60}, {"Red"=227, "Green"=100, "Blue"=56}, {"Red"=229, "Green"=102, "Blue"=52}, {"Red"=231, "Green"=104, "Blue"=48}, {"Red"=233, "Green"=106, "Blue"=44}, {"Red"=235, "Green"=108, "Blue"=40}, {"Red"=237, "Green"=110, "Blue"=36}, {"Red"=239, "Green"=112, "Blue"=32}, {"Red"=241, "Green"=114, "Blue"=28}, {"Red"=243, "Green"=116, "Blue"=24}, {"Red"=245, "Green"=118, "Blue"=20}, {"Red"=247, "Green"=120, "Blue"=16}, {"Red"=249, "Green"=122, "Blue"=12}, {"Red"=251, "Green"=124, "Blue"=8}, {"Red"=253, "Green"=126, "Blue"=4}, {"Red"=255, "Green"=128, "Blue"=0}, {"Red"=255, "Green"=130, "Blue"=4}, {"Red"=255, "Green"=132, "Blue"=8}, {"Red"=255, "Green"=134, "Blue"=12}, {"Red"=255, "Green"=136, "Blue"=16}, {"Red"=255, "Green"=138, "Blue"=20}, {"Red"=255, "Green"=140, "Blue"=24}, {"Red"=255, "Green"=142, "Blue"=28}, {"Red"=255, "Green"=144, "Blue"=32}, {"Red"=255, "Green"=146, "Blue"=36}, {"Red"=255, "Green"=148, "Blue"=40}, {"Red"=255, "Green"=150, "Blue"=45}, {"Red"=255, "Green"=152, "Blue"=49}, {"Red"=255, "Green"=154, "Blue"=53}, {"Red"=255, "Green"=156, "Blue"=57}, {"Red"=255, "Green"=158, "Blue"=61}, {"Red"=255, "Green"=160, "Blue"=65}, {"Red"=255, "Green"=162, "Blue"=69}, {"Red"=255, "Green"=164, "Blue"=73}, {"Red"=255, "Green"=166, "Blue"=77}, {"Red"=255, "Green"=168, "Blue"=81}, {"Red"=255, "Green"=170, "Blue"=85}, {"Red"=255, "Green"=172, "Blue"=89}, {"Red"=255, "Green"=174, "Blue"=93}, {"Red"=255, "Green"=176, "Blue"=97}, {"Red"=255, "Green"=178, "Blue"=101}, {"Red"=255, "Green"=180, "Blue"=105}, {"Red"=255, "Green"=182, "Blue"=109}, {"Red"=255, "Green"=184, "Blue"=113}, {"Red"=255, "Green"=186, "Blue"=117}, {"Red"=255, "Green"=188, "Blue"=121}, {"Red"=255, "Green"=190, "Blue"=125}, {"Red"=255, "Green"=193, "Blue"=130}, {"Red"=255, "Green"=195, "Blue"=134}, {"Red"=255, "Green"=197, "Blue"=138}, {"Red"=255, "Green"=199, "Blue"=142}, {"Red"=255, "Green"=201, "Blue"=146}, {"Red"=255, "Green"=203, "Blue"=150}, {"Red"=255, "Green"=205, "Blue"=154}, {"Red"=255, "Green"=207, "Blue"=158}, {"Red"=255, "Green"=209, "Blue"=162}, {"Red"=255, "Green"=211, "Blue"=166}, {"Red"=255, "Green"=213, "Blue"=170}, {"Red"=255, "Green"=215, "Blue"=174}, {"Red"=255, "Green"=217, "Blue"=178}, {"Red"=255, "Green"=219, "Blue"=182}, {"Red"=255, "Green"=221, "Blue"=186}, {"Red"=255, "Green"=223, "Blue"=190}, {"Red"=255, "Green"=225, "Blue"=194}, {"Red"=255, "Green"=227, "Blue"=198}, {"Red"=255, "Green"=229, "Blue"=202}, {"Red"=255, "Green"=231, "Blue"=206}, {"Red"=255, "Green"=233, "Blue"=210}, {"Red"=255, "Green"=235, "Blue"=215}, {"Red"=255, "Green"=237, "Blue"=219}, {"Red"=255, "Green"=239, "Blue"=223}, {"Red"=255, "Green"=241, "Blue"=227}, {"Red"=255, "Green"=243, "Blue"=231}, {"Red"=255, "Green"=245, "Blue"=235}, {"Red"=255, "Green"=247, "Blue"=239}, {"Red"=255, "Green"=249, "Blue"=243}, {"Red"=255, "Green"=251, "Blue"=247}, {"Red"=255, "Green"=253, "Blue"=251}, {"Red"=255, "Green"=255, "Blue"=255}]  # User Palette
    }
  }
  "error out" <- w3
  "User Palette" <- w1
